vi "Configure Temperature.vi"(8 "error in (no error)":errorcluster, 10 "Temperature [degC]":dbl, 11 "Temperature Control in":refnum<class "Temperature Control.lvclass">) -> (0 "error out":errorcluster, 3 "Temperature Control out":refnum<class "Temperature Control.lvclass">)   [LabVIEW 2020, in "Temperature Control.lvclass"]
uses:
  Temperature Control.lvclass
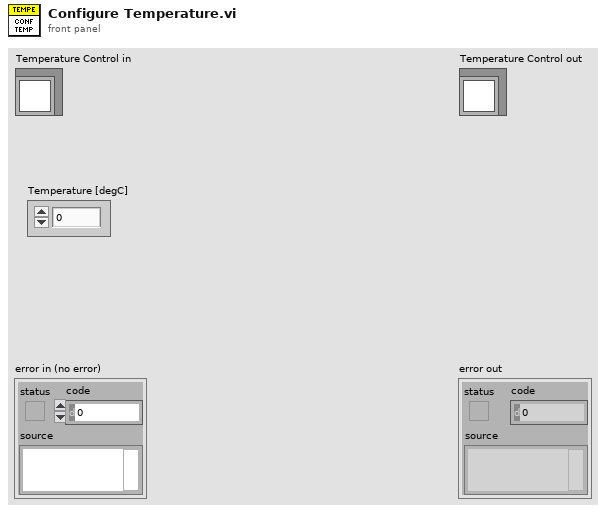
[diagram p1: front panel]
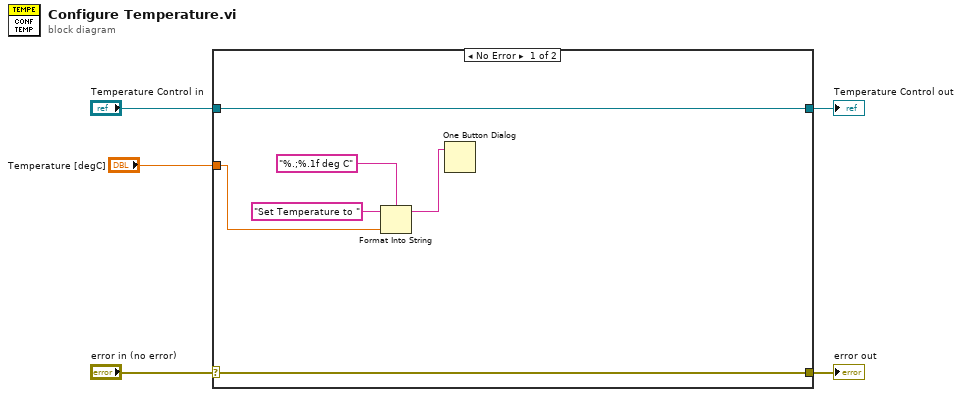
[diagram p0: block diagram]
diagram:
  n1 = case shown="No Error" "error in (no error)" {
    selector: "error in (no error)" -> [w10 w13]
    tunnel: [w10 w13] -> w4
    tunnel: [w11 w12] -> w2
    tunnel: "Temperature Control in" -> [w11 w12]
    tunnel: "Temperature [degC]" -> [w6 _]
    frame No Error {
      n2 = Format Into String(format string="%.;%.1f deg C", initial string="Set Temperature to ", w6) -> (resulting string=w7:string)  [unwired: 1 in, 1 out]
      n3 = One Button Dialog(message=w7) -> ()  [unwired: 1 in, 1 out]
    }
    frame Error {
    }
  }
  "error out" <- w4
  "Temperature Control out" <- w2
